vi "GetOpenSRs.vi"(6 "error in (no error)":errorcluster, 8 "SRs Array":T1[](array[typedef])) -> (0 "error out":errorcluster, 2 "Open SRs":T1[](array[typedef]))   [LabVIEW 2017, in "DS_Lib.lvlib" / "SRReportParser.lvlib"]
uses:
  TypeDefs/InWorkSR_Data.ctl
  SRReportParser.lvlib
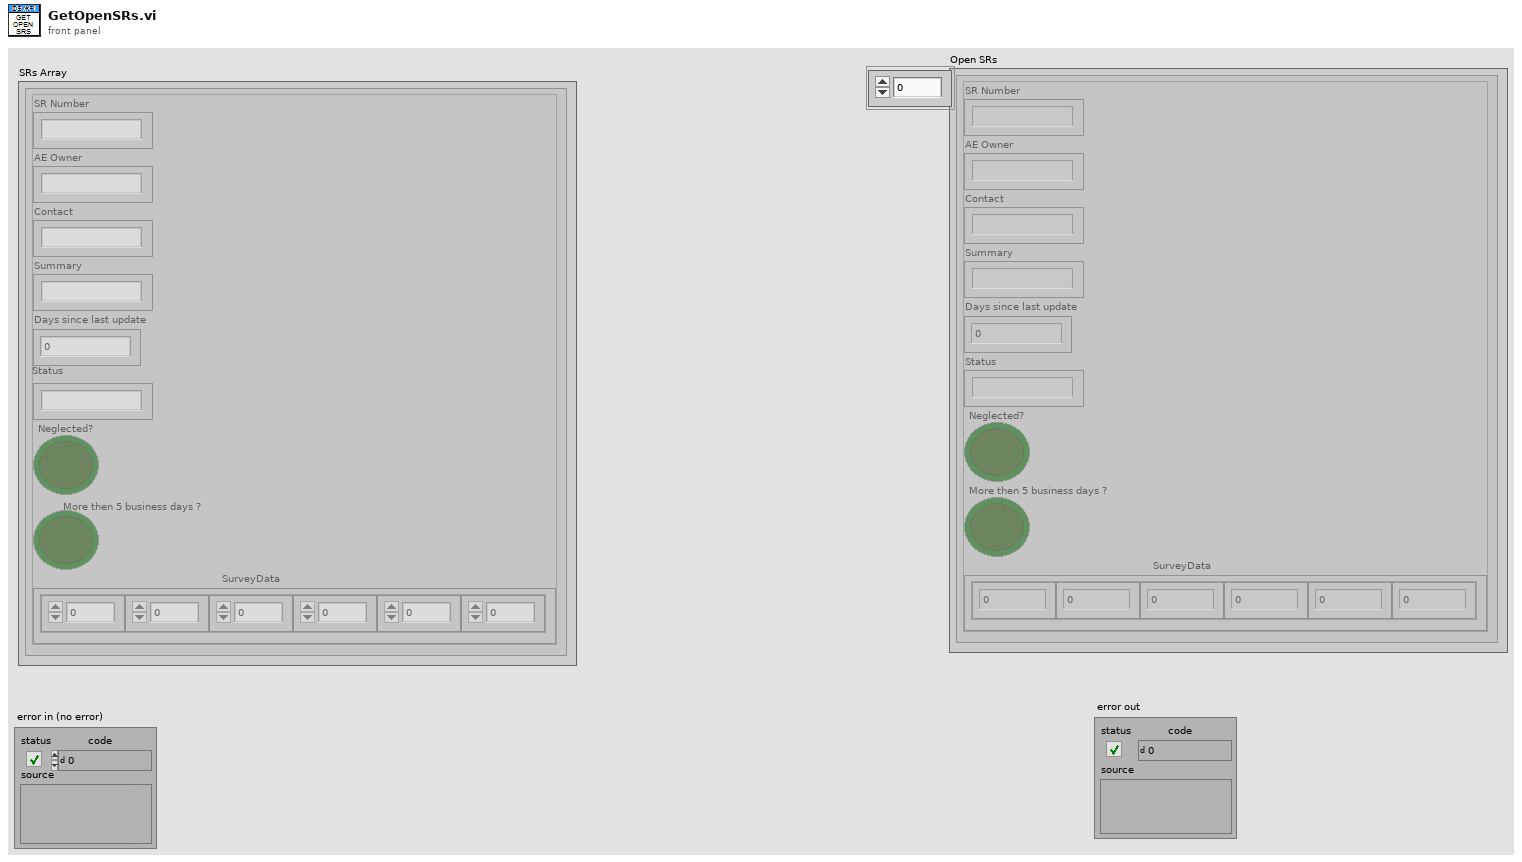
[diagram p1: front panel]
types:
  T1 = typedef "DS_Lib.lvlib/SRReportParser.lvlib/InWorkSR_Data.ctl" = cluster{"SR Number":string, "AE Owner":string, "Contact":string, "Summary":string, "Days since last update":dbl, "Status":string, "Neglected?":bool, "More then 5 business days ?":bool, "SurveyData":cluster{"Resolution Time":dbl, "Total Satisfaction":dbl, "Response Time":dbl, "Courtesy":dbl, "Problem Solved":dbl, "Level of effort":dbl}}
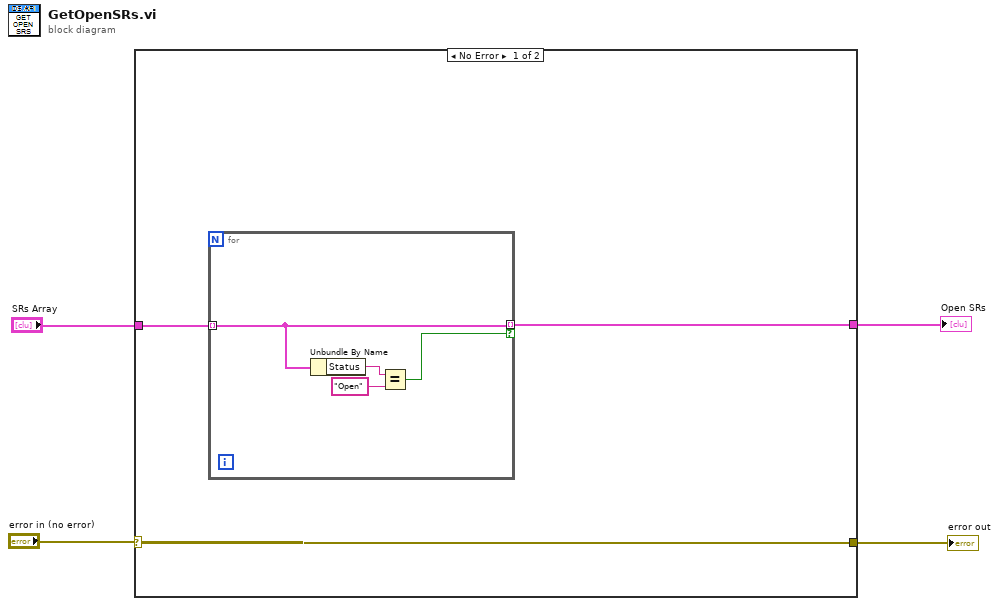
[diagram p0: block diagram]
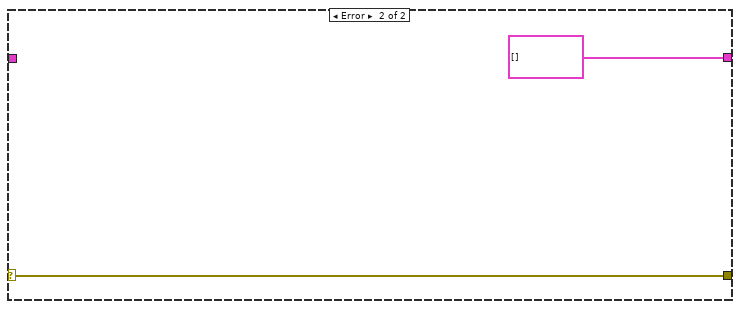
[diagram p2: hidden frame]
diagram:
  n1 = case shown="No Error" "error in (no error)" {
    selector: "error in (no error)" -> [w7 w12]
    tunnel: [w7 w12] -> w3
    tunnel: "SRs Array" -> [w6 _]
    tunnel: [w5 T1[] []] -> w1
    frame No Error {
      n2 = for {
        tunnel: w6 -> [w11] mode=indexing
        tunnel: [w11] -> w5 mode=indexing if=w8
        n3 = Unbundle By Name(w11) -> ("Status"=w10:string)
        n4 = Equal?(x=w10, y="Open") -> (x = y?=w8:bool)
      }
    }
    frame Error {
    }
  }
  "error out" <- w3
  "Open SRs" <- w1
